vi "Error 5023.vi"(8 "error in (no error)":errorcluster, 10 "Additional Error text":string) -> (0 "error out":errorcluster)   [LabVIEW 2019, in "gRPC Template Creation Utility.lvlib"]
uses:
  gRPC Template Creation Utility.lvlib
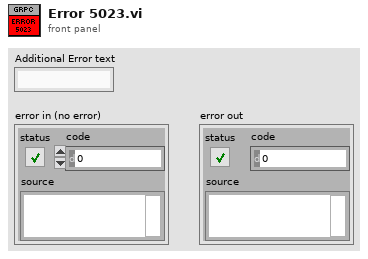
[diagram p1: front panel]
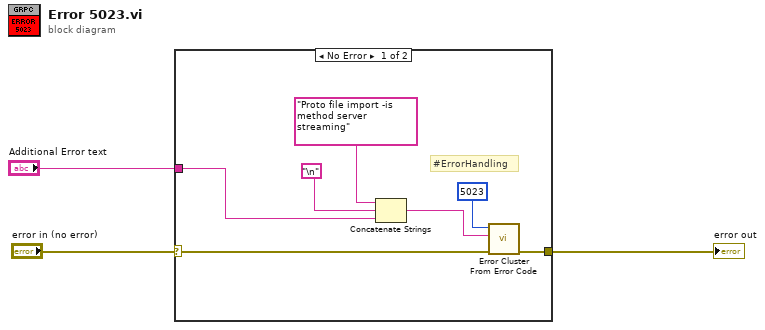
[diagram p0: block diagram]
diagram:
  n1 = case shown="No Error" "error in (no error)" {
    selector: "error in (no error)" -> [w4 w11]
    tunnel: [w10 w11] -> w3
    tunnel: "Additional Error text" -> [w8 _]
    frame No Error {
      # "#ErrorHandling"
      n2 = Concatenate Strings("Proto file import -is method server streaming" ("error message (\"\")"), "\n", w8) -> (w9:string)
      n3 = call <vilib>:"Error Cluster From Error Code.vi"("error in (no error)"=w4, "error message (\"\")"=w9, "error code (0)"=5023) -> ("error out"=w10:errorcluster)  [unwired: 6 in]
    }
    frame Error {
    }
  }
  "error out" <- w3
